vi "Test Split Text into Words.vi"(11 "Test Case In":refnum<class "Text-Based VI Icon Tests.lvclass">) -> (0 "error out":errorcluster, 3 "Test Case Out":refnum<class "Text-Based VI Icon Tests.lvclass">)   [LabVIEW 2020, in "Text-Based VI Icon Tests.lvclass"]
doc: "Contains all the tests related to the function Split Text to Words"
uses:
  Text-Based VI Icon Tests.lvclass
  Text-Based VI Icon Tests.lvclass/Text-Based VI Icon Tests.ctl
  vi.lib/LabVIEW Icon API/Set Text Icon/Text-Based VI Icon.lvlib
  b701d854-ee88-4139-aee6-e1b35b6e74f0.vi
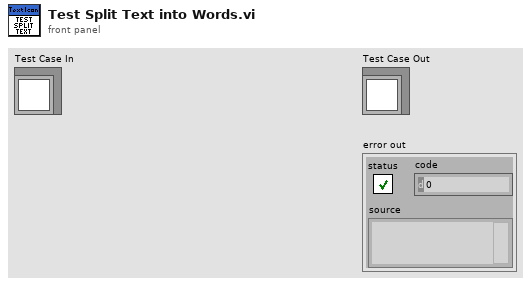
[diagram p1: front panel]
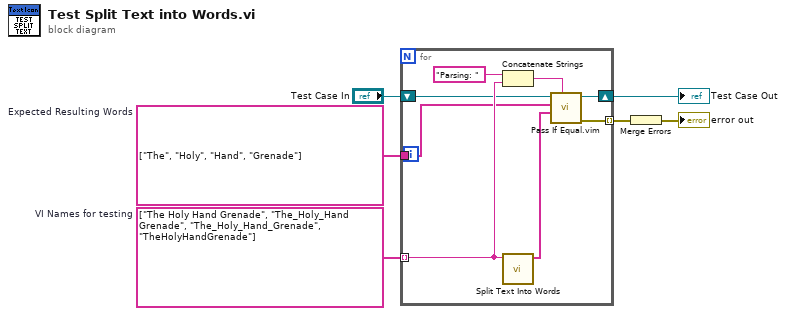
[diagram p0: block diagram]
diagram:
  w4 = string[] ["The", "Holy", "Hand", "Grenade"]  # Expected Resulting Words
  w5 = string[] ["The Holy Hand Grenade", "The_Holy_Hand Grenade", "The_Holy_Hand_Grenade", "TheHolyHandGrenade"]  # VI Names for testing
  n1 = for {
    tunnel: w5 -> [w13] mode=indexing
    tunnel: [w14] -> w3 mode=indexing
    tunnel: w4 -> [w9]
    shift-right: [w10] -> w1
    shift-left: "Test Case In" -> [w7]
    n2 = Concatenate Strings("Parsing: ", w13) -> (w11:string)
    n3 = call "Split Text Into Words.vi"("VI Name"=w13) -> ("Array"=w8:string[])  [unwired: 10 in]
    n4 = call "Pass If Equal.vim"("Description"=w11, "Actual"=w8, "Expected"=w9, "LUnit Test Case In"=w7) -> ("error out"=w14:errorcluster, "LUnit Test Case Out"=w10:refnum<class "Text-Based VI Icon Tests.lvclass">)  [unwired: 6 in]
  }
  "Test Case Out" <- w1
  n5 = Merge Errors(w3) -> (→"error out":errorcluster)
